vi "Hardware - NI 9757-1 (O2) Host.vi"() -> ()   [LabVIEW 2015, in "ECS-Host.lvlib"]
uses:
  ECS-Host.lvlib
panel:
  in  "UEGO2Range":bool
  in  "UEGO1Range":bool
  out "FPGAInterfaceError":bool
  in  "CombustionMode":enum32{"a", "b"}(ring)
  in  "UEGOFilter":sgl caption="[V]"
  out "UEGO2HeaterDutyCycle":sgl caption="[%]"
  in  "UEGO2BackPressure_Man":sgl caption="[bar]"
  in  "UEGO2BackPressure_ManE":bool
  out "UEGO2BackPressure":sgl caption="[bar]"
  out "UEGO2SensorFault":enum32{"NO FAULT", "SHORT TO GND OR BATT"}(ring)
  out "UEGO2Ip":sgl caption="[mA]"
  out "UEGO2AFRatio":sgl
  out "UEGO2Phi":sgl
  out "UEGO2Lambda":sgl
  out "UEGO2HeaterFault":T1(ring)
  out "UEGO2Temp":sgl caption="[F]"
  in  "UEGO2_E":bool
  out "UEGO2Hot":bool
  out "UEGO1HeaterDutyCycle":sgl caption="[%]"
  in  "UEGO1BackPressure_Man":sgl caption="[bar]"
  in  "UEGO1BackPressure_ManE":bool
  out "UEGO1BackPressure":sgl caption="[bar]"
  out "UEGO1SensorFault":enum32{"NO FAULT", "SHORT TO GND OR BATT"}(ring)
  out "UEGO1Ip":sgl caption="[mA]"
  out "UEGO1AFRatio":sgl
  out "UEGO1Phi":sgl
  out "UEGO1Lambda":sgl
  out "UEGO1HeaterFault":T1(ring)
  out "UEGO1Temp":sgl caption="[F]"
  in  "UEGO1_E":bool
  out "UEGO1Hot":bool
  out "FuseStatus":enum32{"FUSE OK", "FUSE BLOWN"}(ring)
  out "EGO4Status":T2(ring)
  in  "EGO4_E":bool
  out "EGO4SensorV":sgl caption="[V]"
  out "EGO3Status":T2(ring)
  in  "EGO3_E":bool
  out "EGO3SensorV":sgl caption="[V]"
  out "EGO2Status":T2(ring)
  in  "EGO2_E":bool
  out "EGO2SensorV":sgl caption="[V]"
  out "EGO1Status":T2(ring)
  in  "EGO1_E":bool
  out "EGO1SensorV":sgl caption="[V]"
  in  "ModuleEnable":bool
  out "Battery":sgl caption="[V]"
  out "ModulePresent":bool
  # "UEGO1"
  # "UEGO2"
  # "Lambda"
  # "Phi"
  # "Lambda"
  # "AFR"
  # "Phi"
  # "AFR"
  # "EGO4"
  # "EGO3"
  # "EGO2"
  # "EGO1"
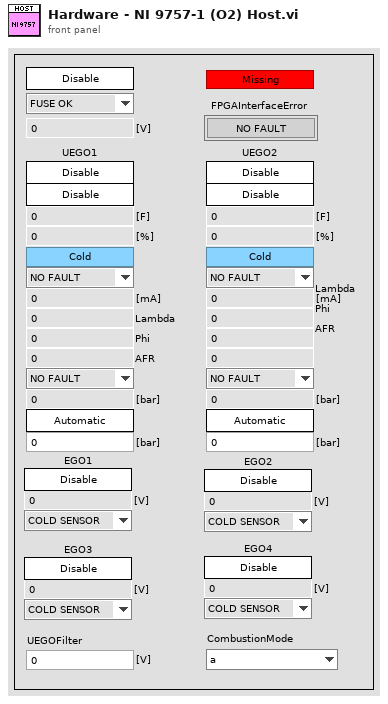
[diagram p1: front panel]
types:
  T1 = enum32{"NO FAULT", "SHORT TO BATTERY", "OPEN CIRCUIT", "SHORT TO GROUND"}
  T2 = enum32{"COLD SENSOR", "FOULED SENSOR", "RICH", "LEAN"}
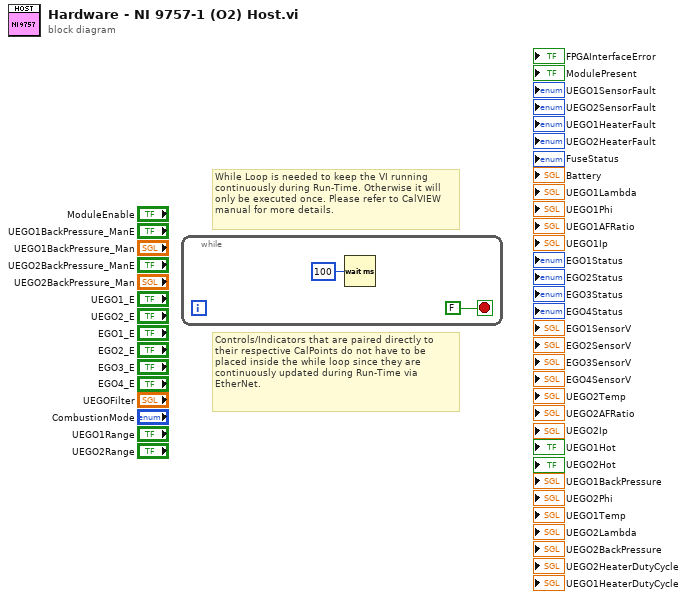
[diagram p0: block diagram]
diagram:
  # "While Loop is needed to keep the VI running\ncontinuously during Run-Time. Otherwise it will only be executed once. Please refer to CalVIEW manual for more details."
  # "Controls/Indicators that are paired directly to their respective CalPoints do not have to be placed inside the while loop since they are continuously updated during Run-Time via EtherNet."
  n1 = while {
    stop <- FALSE stop-if-true
    n2 = Wait (ms)(milliseconds to wait=u32 100) -> ()  [unwired: 1 out]
  }
